vi "Experiment_Settings_Live.vi"() -> ()   [LabVIEW 2013]
uses:
  <userlib>/Accelerator/User Interface/Controls/DisplayExperimentSetting.ctl
panel:
  in  "stop":bool
  in  "small?":bool
  out "error out":errorcluster
  in  "error in (no error)":errorcluster
  out "Experiment Settings":T1
  # "Experiment Status:"
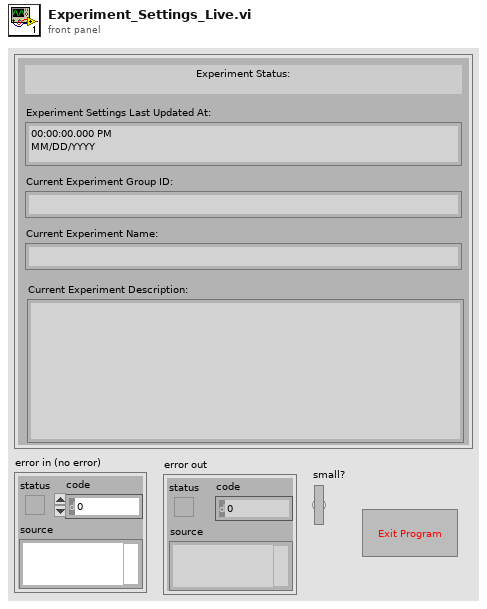
[diagram p1: front panel]
types:
  T1 = typedef "DisplayExperimentSetting.ctl" = cluster{"Current Experiment Name:":string, "Current Experiment Description:":string, "Current Experiment Group ID:":string, "Experiment Settings Last Updated At:":timestamp}
  T2 = typedef "LVRectTypeDef.ctl" = cluster{"Left":i16, "Top":i16, "Right":i16, "Bottom":i16}
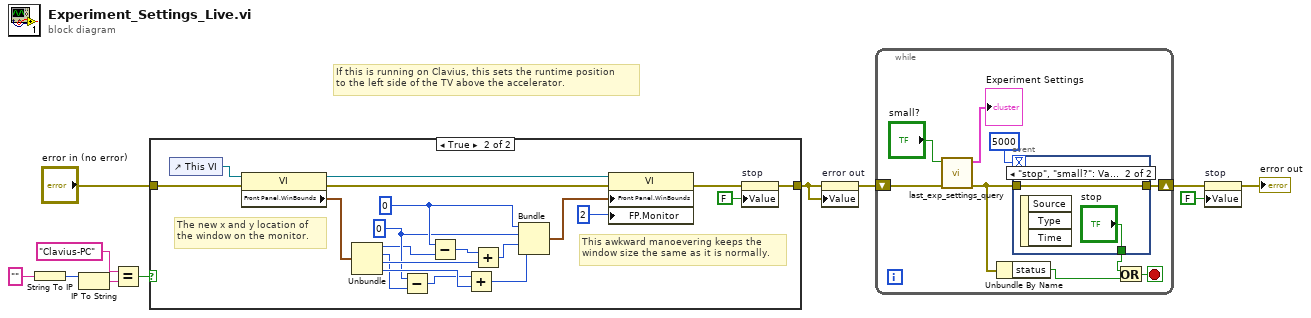
[diagram p0: block diagram]
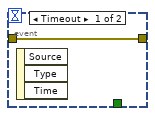
[diagram p3: hidden frame]
diagram:
  # "If this is running on Clavius, this sets the runtime position\nto the left side of the TV above the accelerator."
  n1 = String To IP(1:"" ("name")) -> (0:w8:u32)
  n2 = IP To String(2:w8) -> (0:w10:string)  [unwired: 1 in]
  n3 = Equal?(x="Clavius-PC", y=w10) -> (x = y?=w6:bool)
  n4 = case shown="True" w6 {
    tunnel: "error in (no error)" -> [w12 w17]
    tunnel: [w12 w14] -> w1
    frame False {
    }
    frame True {
      w22 = i16 0 ("Top")
      w23 = i16 0 ("Left")
      # "This awkward manoevering keeps the\nwindow size the same as it is normally."
      # "The new x and y location of\nthe window on the monitor."
      n5 = control-ref of="This VI"() -> (w31:refnum<vi>)
      n6 = property class="VI"(reference=w31, error in=w17) -> (reference out=w27:refnum<vi>, error out=w16:errorcluster, "Front Panel.WinBounds"=w26:T2)
      n7 = Unbundle(w26) -> ("Left"=w21:i16, "Top"=w20:i16, "Right"=w25:i16, "Bottom"=w24:i16)
      n8 = Subtract(x=w22, y=w20) -> (x-y=w19:i16)
      n9 = Subtract(x=w23, y=w21) -> (x-y=w18:i16)
      n10 = Add(x=w19, y=w24) -> (x+y=w28:i16)
      n11 = Add(x=w18, y=w25) -> (x+y=w29:i16)
      n12 = Bundle("Left"=w23, "Top"=w22, w29, w28) -> (w32:cluster{"Left":i16, "Top":i16, i16, i16})  [unwired: 1 in]
      n13 = property class="VI"(reference=w27, error in=w16, "Front Panel.WinBounds"=w32, "FP.Monitor"=u16 2 ("Front Panel Window:Monitor")) -> (error out=w13:errorcluster)  [unwired: 1 out]
      n14 = property on="stop" class="Bool (strict)"(error in=w13, "Value"=FALSE ("stop")) -> (error out=w14:errorcluster)  [unwired: 1 in, 1 out]
    }
  }
  n15 = property on="error out" class="Clust (strict)"(error in=w1, "Value"=w1) -> (error out=w2:errorcluster)  [unwired: 1 in, 1 out]
  n16 = while {
    shift-right: [w41] -> w11
    shift-left: w2 -> [w36]
    stop <- w39 stop-if-true
    n17 = call <userlib>:"last_exp_settings_query.vi"("error in (no error)"=w36, "Small?"="small?") -> ("error out"=w34:errorcluster, "Experiment Settings"=→"Experiment Settings":T1)  [unwired: 4 in, 4 out]
    n18 = Unbundle By Name(w34) -> ("status"=w37:bool)
    n19 = event shown="[1] \"stop\", \"small?\": Value Change" {
      selector: _ -> [_ _]
      dyn-events: _ -> [_ _]
      timeout: u32 5000 ("milliseconds to wait") -> [_ _]
      tunnel: w34 -> [w42 w43]
      tunnel: [w42 w43] -> w41
      tunnel: [_ "stop"] -> w38
      event Timeout {
        n20 = event-data() -> ()  [unwired: 1 in, 3 out]
      }
      event "stop", "small?": Value Change {
        n21 = event-data() -> ()  [unwired: 1 in, 3 out]
      }
    }
    n22 = Or(x=w38, y=w37) -> (x .or. y?=w39:bool)
  }
  n23 = property on="stop" class="Bool (strict)"(error in=w11, "Value"=FALSE ("stop")) -> (error out=→"error out":errorcluster)  [unwired: 1 in, 1 out]
